vi "dfd_Get Cosine Matrix.vi"(6 "w":dbl, 8 "error in (no error)":errorcluster, 10 "order":i32, 11 "number of bands":i32) -> (0 "error out":errorcluster, 2 "CT":dbl[][](array[numeric]), 3 "C":dbl[][](array[numeric]))   [LabVIEW 2017, in "NI_DigFilter_FilterBank.lvlib"]
uses:
  <vilib>/addons/Digital Filter Design/NI_DigFilter_FilterBank.lvlib
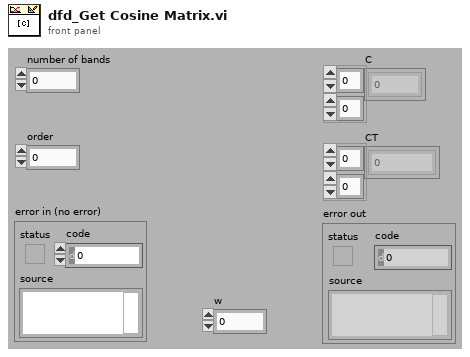
[diagram p1: front panel]
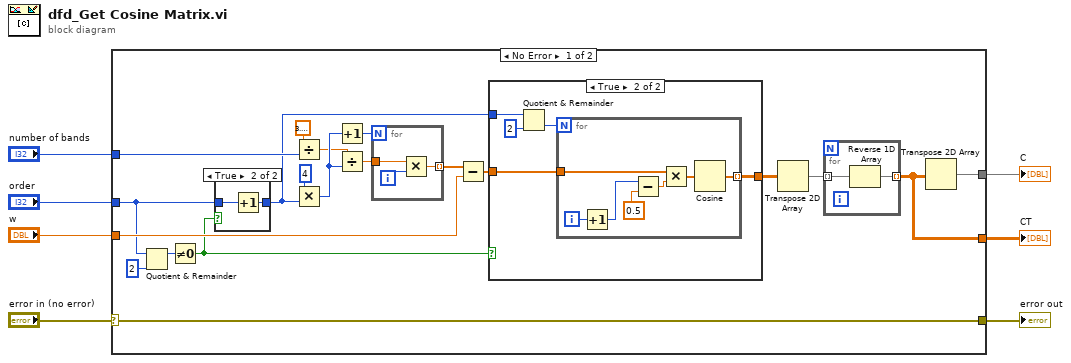
[diagram p0: block diagram]
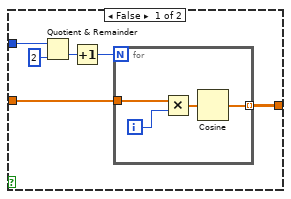
[diagram p3: hidden frame]
diagram:
  n1 = case shown="No Error" "error in (no error)" {
    selector: "error in (no error)" -> [w8 w58]
    tunnel: [w27 _] -> w7
    tunnel: "number of bands" -> [w21 _]
    tunnel: "w" -> [w16 _]
    tunnel: "order" -> [w13 _]
    tunnel: [w10 _] -> w3
    tunnel: [w8 w58] -> w2
    frame No Error {
      n2 = Quotient & Remainder(x=w13, y=2) -> (x-y*floor(x/y)=w11:i32)  [unwired: 1 out]
      n3 = Not Equal To 0?(x=w11) -> (x != 0?=w9:bool)
      n4 = case shown="True" w9 {
        tunnel: w13 -> [w28 w30]
        tunnel: [w28 w29] -> w14
        frame False {
        }
        frame True {
          n5 = Increment(x=w30) -> (x+1=w29:i32)
        }
      }
      n6 = Divide(x=3.141592653589793, y=w21) -> (x/y=w22:dbl)
      n7 = Multiply(x=4, y=w14) -> (x*y=w24:i32)
      n8 = Increment(x=w24) -> (x+1=w25:i32)
      n9 = Divide(x=w22, y=w24) -> (x/y=w23:dbl)
      n10 = for {
        N: w25 -> [_]
        tunnel: w23 -> [w56]
        tunnel: [w55] -> w17 mode=indexing
        i -> [w57]
        n11 = Multiply(x=w56, y=w57) -> (x*y=w55:dbl)
      }
      n12 = Subtract(x=w17, y=w16) -> (x-y=w18:dbl[])
      n13 = case shown="True" w9 {
        tunnel: [w36 w41] -> w26
        tunnel: w18 -> [w35 w42]
        tunnel: w14 -> [w33 w43]
        frame False {
          n14 = Quotient & Remainder(x=w33, y=2) -> (floor(x/y)=w32:i32)  [unwired: 1 out]
          n15 = Increment(x=w32) -> (x+1=w31:i32)
          n16 = for {
            N: w31 -> [_]
            tunnel: w35 -> [w40]
            tunnel: [w39] -> w36 mode=indexing
            i -> [w37]
            n17 = Multiply(x=w40, y=w37) -> (x*y=w38:dbl[])
            n18 = Cosine(x=w38) -> (cos(x)=w39:dbl[])
          }
        }
        frame True {
          n19 = Quotient & Remainder(x=w43, y=2) -> (floor(x/y)=w44:i32)  [unwired: 1 out]
          n20 = for {
            N: w44 -> [_]
            tunnel: w42 -> [w52]
            tunnel: [w49] -> w41 mode=indexing
            i -> [w51]
            n21 = Increment(x=w51) -> (x+1=w50:i32)
            n22 = Subtract(x=w50, y=0.5) -> (x-y=w47:dbl)
            n23 = Multiply(x=w52, y=w47) -> (x*y=w46:dbl[])
            n24 = Cosine(x=w46) -> (cos(x)=w49:dbl[])
          }
        }
      }
      n25 = Transpose 2D Array(2D array=w26) -> (transposed array=w15:dbl[][])
      n26 = for {
        tunnel: w15 -> [w54] mode=indexing
        tunnel: [w53] -> w10 mode=indexing
        n27 = Reverse 1D Array(array=w54) -> (reversed array=w53:dbl[])
      }
      n28 = Transpose 2D Array(2D array=w10) -> (transposed array=w27:dbl[][])
    }
    frame Error {
    }
  }
  "C" <- w7
  "CT" <- w3
  "error out" <- w2
